vi "GPS Compass.vi"(1 "Compass Longitude 2":dbl format="%_16g", 2 "Compass Latitude 2":dbl format="%_16g", 3 "Compass Longitude 1":dbl, 4 "Compass Latitude 1":dbl) -> (0 "Compass":dbl)   [LabVIEW 2011]
uses:
  <vilib>/express/express arith-compare/Formula/XNode/ExpressFormulaBlockNode.xnode
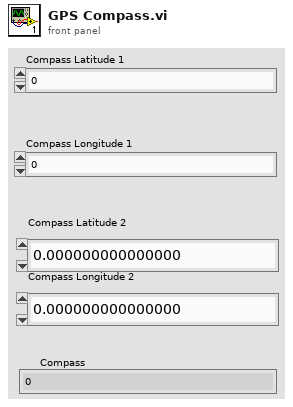
[diagram p1: front panel]
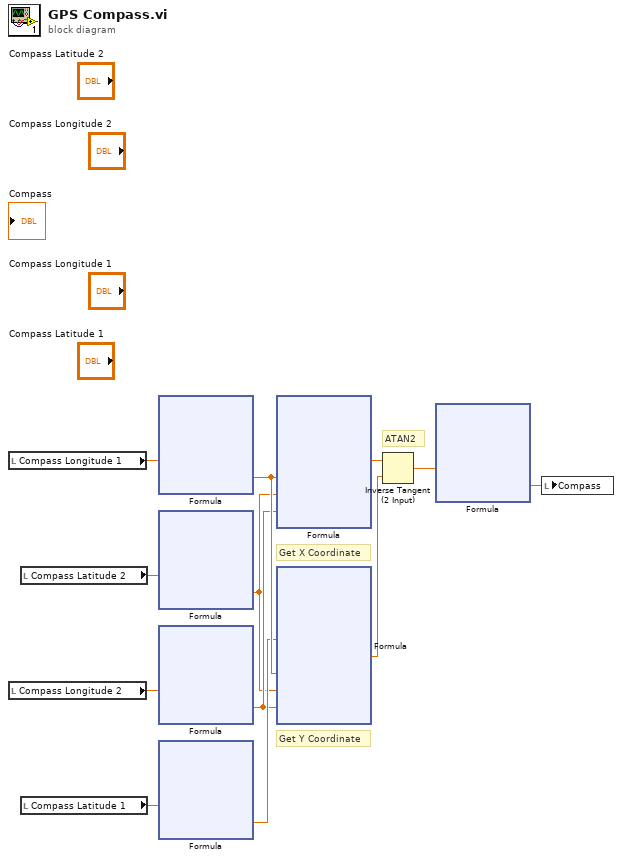
[diagram p0: block diagram]
diagram:
  # "Get X Coordinate"
  # "ATAN2"
  # "Get Y Coordinate"
  n1 = local read "Compass Longitude 1"() -> (w1:dbl)
  n2 = local read "Compass Longitude 2"() -> (w3:dbl)
  n3 = local read "Compass Latitude 2"() -> (w4:dbl)
  n4 = local read "Compass Latitude 1"() -> (w2:dbl)
  n5 = xnode "Formula"("Dlong1"=w1) -> ("Result"=w12:dbl)  [unwired: 1 in, 1 out]
  n6 = xnode "Formula"("Dlat1"=w4) -> ("Result"=w6:dbl)  [unwired: 1 in, 1 out]
  n7 = xnode "Formula"("Dlong1"=w3) -> ("Result"=w7:dbl)  [unwired: 1 in, 1 out]
  n8 = xnode "Formula"("Dlat1"=w2) -> ("Result"=w11:dbl)  [unwired: 1 in, 1 out]
  n9 = xnode "Formula"("PreLong"=w12, "CurLat"=w6, "CurLong"=w7) -> ("Result"=w10:dbl)  [unwired: 1 in, 1 out]
  n10 = xnode "Formula"("PreLat"=w11, "PreLong"=w12, "CurLat"=w6, "CurLong"=w7) -> ("Result"=w9:dbl)  [unwired: 1 in, 1 out]
  n11 = Inverse Tangent (2 Input)(1:w9, 2:w10) -> (0:w8:dbl)
  n12 = xnode "Formula"("rad"=w8) -> ("Result"=w5:dbl)  [unwired: 1 in, 1 out]
  n13 = local write "Compass"(w5) -> ()
